vi "UnlockECU.Compile.vi"(8 "error in (no error)":errorcluster, 11 "Section Ref in":T6 format="%.0x") -> (0 "error out":errorcluster, 1 "Security":T1={"Type"=enum."None", "Source DLL Path"=path "", "Target DLL Path"=path "", "Security Level"=1}, 2 "Settings":T3[](array[typedef]) {"Signal.Cmd.Refs"."Signal Refs" format="%.0x"; "Signal.Cmd.Info"."Signals"."Byte Order" items=["Little Endian", "Big Endian"]; "Signal.Cmd.Info"."Signals"."Data Type" items=["Signed", "Unsigned", "IEEE Float"]; "Settings.Refs"."Signal Refs" format="%.0x"; "Signal.Resp.Refs"."Signal Refs" format="%.0x"; "Signal.Resp.Info"."Signals"."Byte Order" items=["Little Endian", "Big Endian"]; "Signal.Resp.Info"."Signals"."Data Type" items=["Signed", "Unsigned", "IEEE Float"]; "Trigger.Refs"."Signal Refs" format="%.0x"; "Status.Refs"."Signal Refs" format="%.0x"}, 3 "Section Ref out":T6 format="%.0x")   [LabVIEW 2019, in "Diagnostics Addon System Explorer.lvlib"]
uses:
  Diagnostics Addon System Explorer.lvlib
  <vilib>/NI VeriStand/Custom Device API/Custom Device Item Ref.ctl
  Types/Service.Export.ctl
  Types/Frame.Ref.ctl
  Shared/Types/Type.ctl
  Shared/Types/Frame.Compile.ctl
  Shared/Types/Signal.ctl
  Shared/Types/Security.ctl
  Shared/Types/Security.Type.ctl
  Types/FG.Action.ctl
  FileDependency.Create.vi
  <vilib>/NI VeriStand/Custom Device Tools/Custom Device Utility Library/NI VeriStand - Search for Item by GUID.vi
  Shared/SubVIs/Constants.vi
  <vilib>/NI VeriStand/Custom Device API/NI VeriStand - Get Item Children.vi
  <vilib>/NI VeriStand/Custom Device Tools/Custom Device Utility Library/NI VeriStand - Search for Item by Name.vi
  <vilib>/NI/NI VeriStand Advanced SysDef API/SysDef API/SysDef.Property.Set.vi
  <vilib>/NI/NI VeriStand Advanced SysDef API/_SubVIs/SysDef.Property.Set.U32.vi
  <vilib>/NI VeriStand/Custom Device API/NI VeriStand - Get Item Property.vi
  <vilib>/NI VeriStand/Custom Device API/Get Item Property (U32).vi
  FileDependency.Get.Target Path.vi
  <vilib>/Utility/MD5Checksum.llb/MD5Checksum File.vi
  <vilib>/NI/NI VeriStand Advanced SysDef API/_SubVIs/SysDef.Property.Set.DependentFile.vi
  <vilib>/NI/NI VeriStand Advanced SysDef API/SysDef API/SysDef.Property.Remove.vi
  <vilib>/NI VeriStand/Custom Device Tools/Custom Device Utility Library/Custom Device Utility Library.lvlib
  <vilib>/NI VeriStand/Custom Device API/Custom Device API.lvlib
  Shared/Diagnostics Addon Shared.lvlib
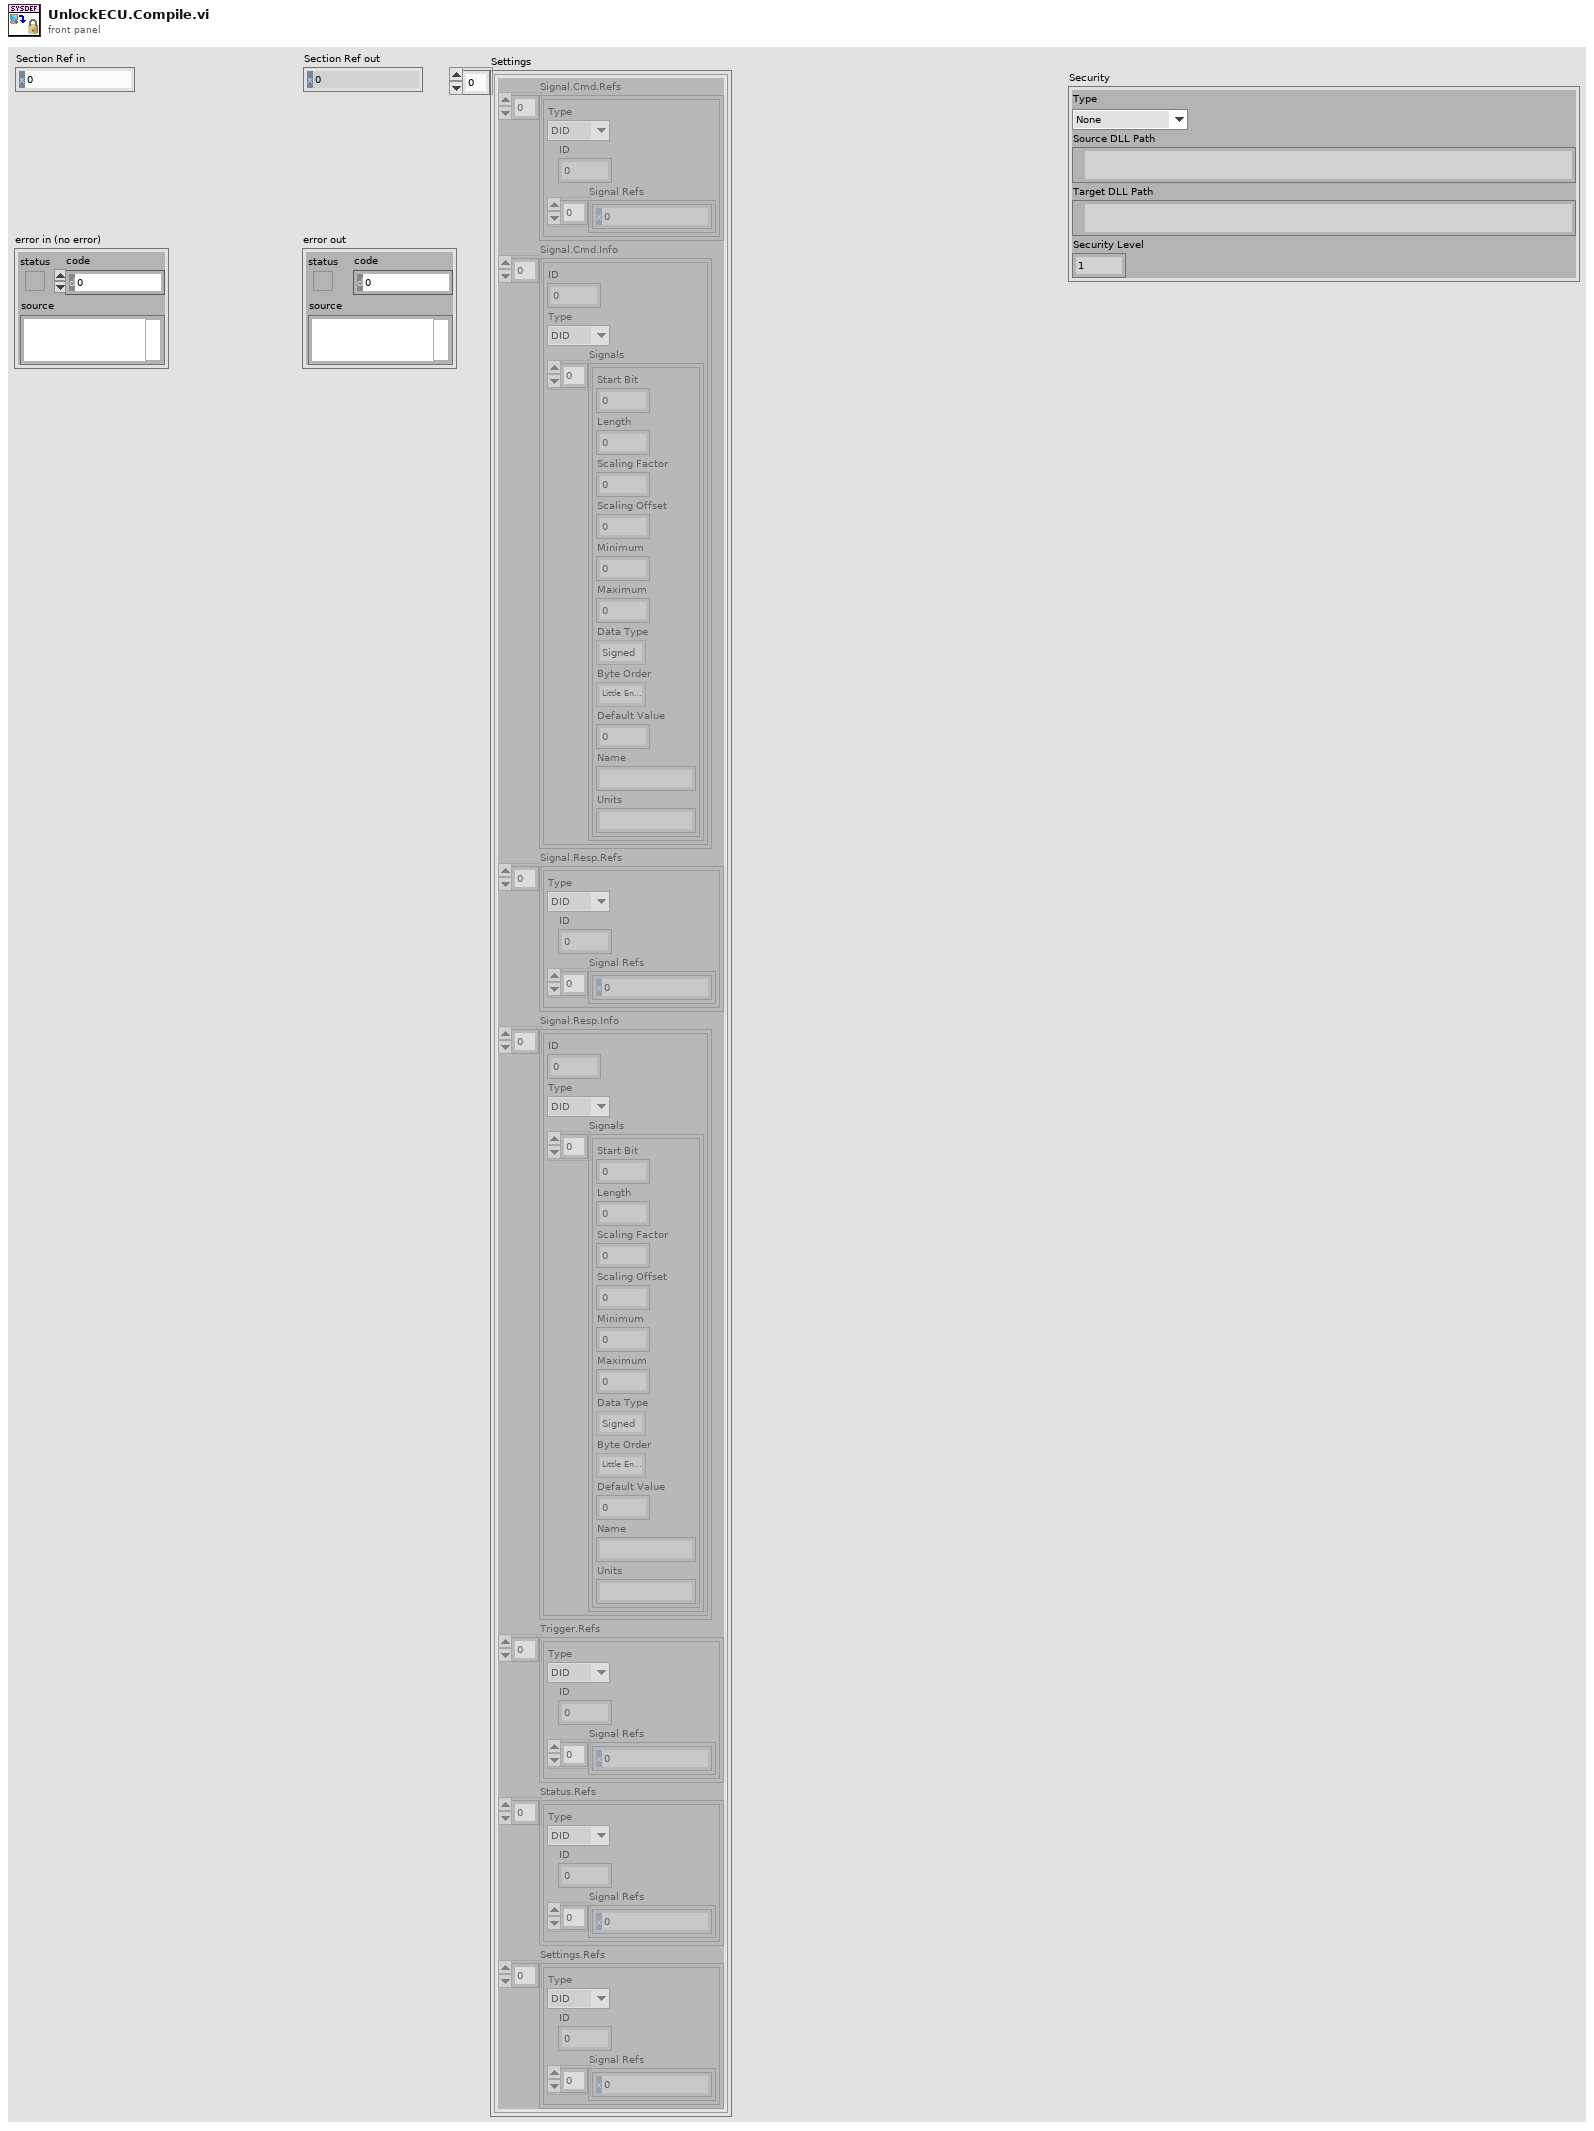
[diagram p1: front panel]
types:
  T1 = typedef "Diagnostics Addon Shared.lvlib/Security.ctl" = cluster{"Type":T2, "Source DLL Path":path, "Target DLL Path":path, "Security Level":u8}
  T2 = typedef "Diagnostics Addon Shared.lvlib/Security.Type.ctl" = enum16{"None", "DLL", "MasterKey"}
  T3 = typedef "Diagnostics Addon System Explorer.lvlib/Service.Export.ctl" = cluster{"Signal.Cmd.Refs":T4[], "Signal.Cmd.Info":T7[], "Signal.Resp.Refs":T4[], "Signal.Resp.Info":T7[], "Trigger.Refs":T4[], "Status.Refs":T4[], "Settings.Refs":T4[]}
  T4 = typedef "Diagnostics Addon System Explorer.lvlib/Frame.Ref.ctl" = cluster{"Type":T5, "ID":u32, "Signal Refs":T6[]}
  T5 = typedef "Diagnostics Addon Shared.lvlib/Type.ctl" = enum16{"DID", "CDID", "PID", "CPID", "Read Memory", "Write Memory", "IO Control", "Routine Start", "Routine Request", "Routine Stop", "User Defined", "DTC Control", "Clear DTCs", "Read DTCs", "Start DTCs", "DTC Change Count", "Tester Present", "Unlock ECU", "Reset ECU", "Diag Session Control", "Communication Control", "DPID Control", "Poll Control", "Diag CAN Control"}
  T6 = typedef "Custom Device API.lvlib/Custom Device Item Ref.ctl" = u64
  T7 = typedef "Diagnostics Addon Shared.lvlib/Frame.Compile.ctl" = cluster{"ID":u32, "Type":T5, "Signals":T8[]}
  T8 = typedef "Diagnostics Addon Shared.lvlib/Signal.ctl" = cluster{"Start Bit":u32, "Length":u32, "Scaling Factor":dbl, "Scaling Offset":dbl, "Minimum":dbl, "Maximum":dbl, "Data Type":u32, "Byte Order":u32, "Default Value":dbl, "Name":string, "Units":string}
  T9 = typedef "Diagnostics Addon System Explorer.lvlib/FG.Action.ctl" = enum16{"Get", "Set"}
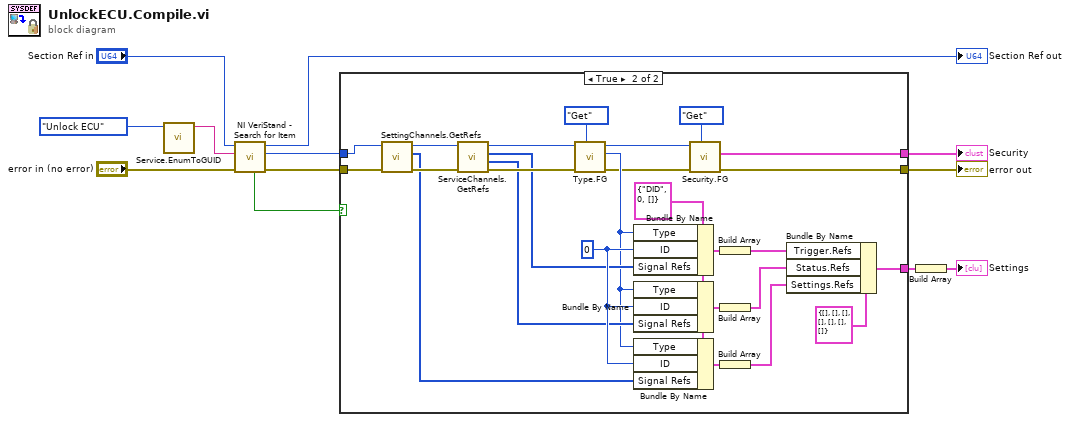
[diagram p0: block diagram]
diagram:
  n1 = call "Service.EnumToGUID.vi"("Type"=Type."Unlock ECU") -> ("GUID"=w4:string)  [unwired: 10 in]
  n2 = call-poly <vilib>:"NI VeriStand - Search for Item.vi"("error in"="error in (no error)", "Item GUID"=w4, "Section Ref in"="Section Ref in") -> ("error out"=w6:errorcluster, "Item Ref"=w7:T6, "Section Ref out"=→"Section Ref out":T6, "Found"=w5:bool)  [unwired: 5 in]
  n3 = case shown="True" w5 {
    tunnel: [w13 w17] -> w9
    tunnel: w7 -> [_ w31]
    tunnel: w6 -> [w13 w33]
    tunnel: [_ w37] -> w8
    tunnel: [_ w14] -> w1
    frame False {
    }
    frame True {
      w27 = 0
      w26 = T4 {"Type"=enum."DID", "ID"=0, "Signal Refs"=[]} ("cluster")
      n4 = call "SettingChannels.GetRefs.vi"("error in (no error)"=w33, "Item Ref in"=w31) -> ("error out"=w36:errorcluster, "Settings"=w23:T6[], "Section Ref out"=w35:T6)  [unwired: 7 in]
      n5 = call "ServiceChannels.GetRefs.vi"("error in (no error)"=w36, "Item Ref in"=w35) -> ("error out"=w34:errorcluster, "Status"=w24:T6[], "Trigger"=w25:T6[], "Section Ref out"=w32:T6)  [unwired: 6 in]
      n6 = call "Type.FG.vi"("Action"=FG.Action."Get", "error in (no error)"=w34, "Device Item Ref in"=w32) -> ("error out"=w18:errorcluster, "Type"=w19:T5, "Device Item Ref out"=w16:T6)  [unwired: 6 in]
      n7 = Bundle By Name(cluster=w26, "Type"=w19, "ID"=w27, "Signal Refs"=w25) -> (w30:T4)
      n8 = Bundle By Name(cluster=w26, "Type"=w19, "ID"=w27, "Signal Refs"=w24) -> (w29:T4)
      n9 = Bundle By Name(cluster=w26, "Type"=w19, "ID"=w27, "Signal Refs"=w23) -> (w28:T4)
      n10 = call "Security.FG.vi"("Action"=FG.Action."Get", "error in (no error)"=w18, "Device Item Ref in"=w16) -> ("error out"=w17:errorcluster, "Security"=w14:T1)  [unwired: 6 in, 1 out]
      n11 = Build Array(w30) -> (w22:T4[])
      n12 = Build Array(w29) -> (w21:T4[])
      n13 = Build Array(w28) -> (w20:T4[])
      n14 = Bundle By Name(cluster=T3 {"Signal.Cmd.Refs"=[], "Signal.Cmd.Info"=[], "Signal.Resp.Refs"=[], "Signal.Resp.Info"=[], "Trigger.Refs"=[], "Status.Refs"=[], "Settings.Refs"=[]}, "Trigger.Refs"=w22, "Status.Refs"=w21, "Settings.Refs"=w20) -> (w37:T3)
    }
  }
  "error out" <- w9
  "Security" <- w1
  n15 = Build Array(w8) -> (→"Settings":T3[])
